vi "CloseNode.vi"(8 "error in":errorcluster, 11 "node ref":T1) -> (0 "error out":errorcluster)   [LabVIEW 2025, in "CEF.lvlib"]
doc: "This is the node Clean Up Vi it will close all the open references for the node and its childs Copyright 2017 National Instruments Corporation\n\nLicensed under the Apache License, Version 2.0 (the \"License\"); you may not use this file except in compliance with the License. You may obtain a copy of the License at http://www.apache.org/licenses/LICENSE-2.0\nUnless required by applicable law or agreed to in writing, software distributed under the License is distributed on an \"AS IS\" BASIS, WITHOUT WARRANTIES OR CONDITIONS OF ANY KIND, either express or implied. See the License for the specific language governing permissions and limitations under the License."
uses:
  CEF.lvlib
  Node/NodeRef.ctl
  Node/CEF_Node.lvclass
  Node/CEF_Node.lvclass/CEF_Node.ctl
  Node/ReadChildren.vi
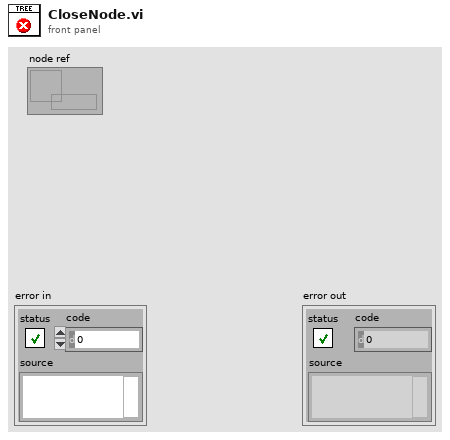
[diagram p1: front panel]
types:
  T1 = typedef "CEF.lvlib/CEF_Node.lvclass/NodeRef.ctl" = refnum<data-value>
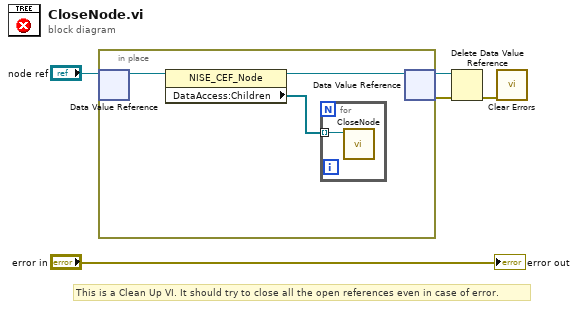
[diagram p0: block diagram]
diagram:
  # "This is a Clean Up VI. It should try to close all the open references even in case of error."
  n1 = in-place {
    n2 = in-place-dvr #1("node ref") -> (w6:refnum<class "CEF_Node.lvclass">)  [unwired: 1 out]
    n3 = property class="NISE_CEF_Node"(reference=w6) -> (reference out=w7:refnum<class "CEF_Node.lvclass">, "DataAccess:Children"=w8:T1[])  [unwired: 1 in, 1 out]
    n4 = for {
      tunnel: w8 -> [w9] mode=indexing
      n5 = call "CloseNode.vi"("node ref"=w9) -> ()  [unwired: 10 in, 1 out]
    }
    n6 = in-place-dvr #1(w7) -> (w4:T1, w2:errorcluster)
  }
  n7 = Delete Data Value Reference(data value reference=w4, error in=w2) -> (error out=w1:errorcluster)  [unwired: 1 out]
  n8 = call <vilib>:"Clear Errors.vi"("error in (no error)"=w1) -> ()  [unwired: 5 in, 2 out]
  "error out" <- "error in"
